vi "Save XML.vi"(8 "error in (no error)":errorcluster, 11 "XML Handler in":refnum<class "XML Handler.lvclass">) -> (0 "error out":errorcluster, 3 "XML Handler out":refnum<class "XML Handler.lvclass">)   [LabVIEW 2020, in "XML Handler.lvclass"]
uses:
  XML Handler.lvclass
  XML Handler.lvclass/XML Handler.ctl
  <resource>/objmgr/DOMUserDefRef.rc
panel:
  out "XML":string
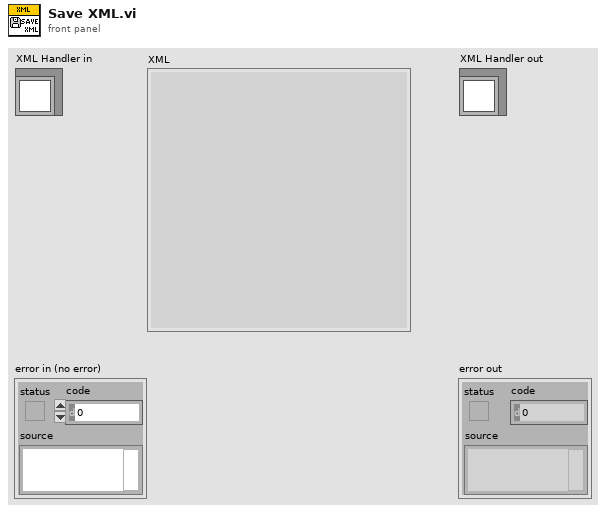
[diagram p1: front panel]
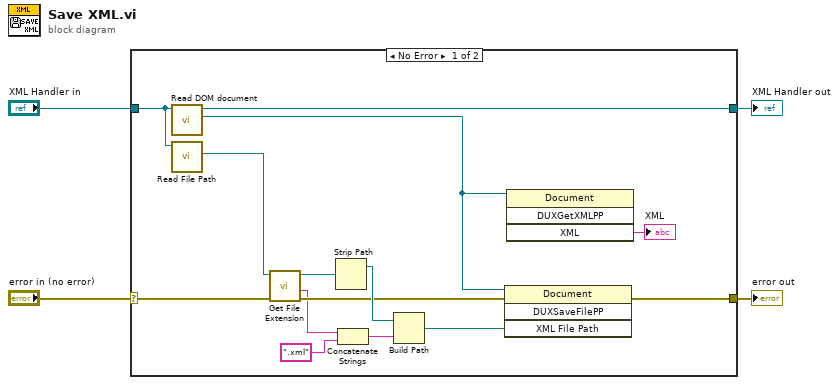
[diagram p0: block diagram]
diagram:
  n1 = case shown="No Error" "error in (no error)" {
    selector: "error in (no error)" -> [w11 w20]
    tunnel: [w16 w20] -> w3
    tunnel: [w18 w19] -> w1
    tunnel: "XML Handler in" -> [w17 w19]
    frame No Error {
      n2 = call "Read DOM document.vi"("XML Handler in"=w17) -> ("DOM document"=w6:refnum<k20>, "XML Handler out"=w18:refnum<class "XML Handler.lvclass">)  [unwired: 9 in]
      n3 = call "Read File Path.vi"("XML Handler in"=w17) -> ("File Path"=w9:path)  [unwired: 9 in, 1 out]
      n4 = call <vilib>:"Get File Extension.vi"("error in (no error)"=w11, "file"=w9) -> ("error out"=w10:errorcluster, "filename without extension"=w7:string, "dup file"=w8:path)  [unwired: 5 in, 2 out]
      n5 = Strip Path(path=w8) -> (stripped path=w14:path)  [unwired: 1 out]
      n6 = Concatenate Strings(w7, ".xml" ("string")) -> (w13:string)
      n7 = Build Path(base path=w14, name or relative path=w13) -> (appended path=w12:path)
      n8 = invoke class="Document" method="DUXSaveFilePP"(reference=w6, error in=w10, "XML File Path"=w12) -> (error out=w16:errorcluster)  [unwired: 1 in, 3 out]
      n9 = invoke class="Document" method="DUXGetXMLPP"(reference=w6) -> ("XML"=→"XML":string)  [unwired: 3 in, 3 out]
    }
    frame Error {
    }
  }
  "error out" <- w3
  "XML Handler out" <- w1
